vi "Untitled 4 (SubVI).vi"(11 "AWG":dbl) -> ()   [LabVIEW 2016]
uses:
  <vilib>/express/express arith-compare/Formula/XNode/ExpressFormulaBlockNode.xnode
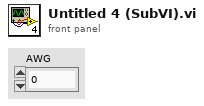
[diagram p1: front panel]
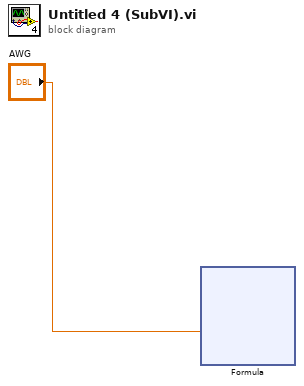
[diagram p0: block diagram]
diagram:
  n1 = xnode "Formula"("X1"="AWG") -> ()  [unwired: 1 in, 2 out]
